vi "DeDuplicateTargets.vi"(1 "TargetsIn":T1[](array[typedef])=[{"Target Type"=0, "Checksum"=0, "Signature Number"=0, "X Center"=0, "Y Center"=0, "Width"=0, "Height"=0, "Angle"=0}] {"Angle" format="%x"; "Height" format="%x"; "Width" format="%x"; "Y Center" format="%x"; "X Center" format="%x"; "Signature Number" format="%x"; "Checksum" format="%x"; "Target Type" items=["PIXY_START_WORD"=43605, "PIXY_START_WORD_CC"=43606, "PIXY_START_WORDX"=21930]}) -> (0 "TargetsOut":T1[](array[typedef]) {"Angle" format="%x"; "Height" format="%x"; "Width" format="%x"; "Y Center" format="%x"; "X Center" format="%x"; "Signature Number" format="%x"; "Checksum" format="%x"; "Target Type" items=["PIXY_START_WORD"=43605, "PIXY_START_WORD_CC"=43606, "PIXY_START_WORDX"=21930]})   [LabVIEW 2016, in "PixyCam_LabVIEW.lvlib"]
uses:
  PixyCam_LabVIEW.lvlib
  PixyCam_TargetData.ctl
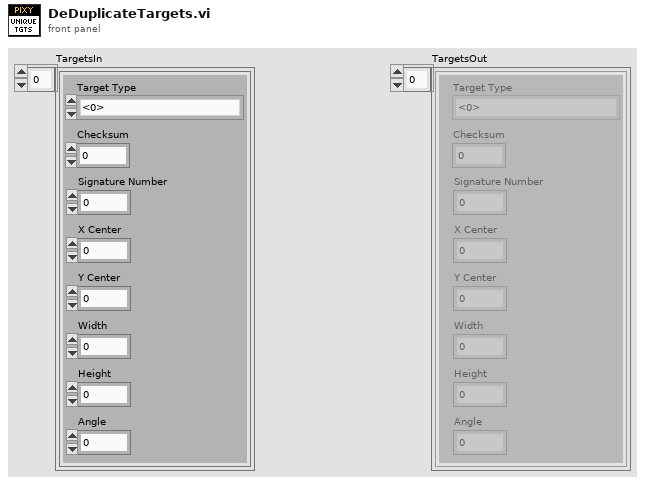
[diagram p1: front panel]
types:
  T1 = typedef "PixyCam_LabVIEW.lvlib/PixyCam_TargetData.ctl" = cluster{"Target Type":u16, "Checksum":u16, "Signature Number":u16, "X Center":u16, "Y Center":u16, "Width":u16, "Height":u16, "Angle":u16}
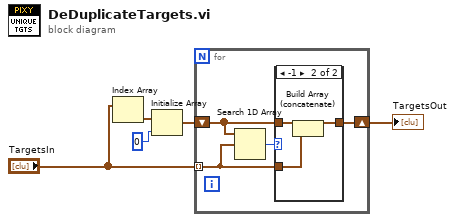
[diagram p0: block diagram]
diagram:
  n1 = Index Array(array="TargetsIn") -> (element=w3:T1)  [unwired: 1 in]
  n2 = Initialize Array(w3, 0 ("Dimension Size")) -> (w4:T1[])
  n3 = for {
    tunnel: "TargetsIn" -> [w8] mode=indexing
    shift-right: [w7] -> w1
    shift-left: w4 -> [w6]
    n4 = Search 1D Array(1D array=w6, element=w8) -> (index of element=w9:i32)  [unwired: 1 in]
    n5 = case shown="-1" w9 {
      tunnel: w8 -> [_ w13]
      tunnel: [w10 w11] -> w7
      tunnel: w6 -> [w10 w12]
      frame Default {
      }
      frame -1 {
        n6 = Build Array (concatenate)(w12, w13) -> (w11:T1[])
      }
    }
  }
  "TargetsOut" <- w1
